vi "Construct Terminal Enabled State Binding.vi"(7 "Initial State (T)":bool=TRUE, 8 "FALSE State (Disabled and Grayed Out)":T1(ring)=enum."Disabled and Grayed Out", 9 "TRUE State (Enabled)":T1(ring), 10 "Control":refnum<vi>) -> (0 "error out":errorcluster, 3 "TerminalEnabledStateBinding":refnum<class "TerminalEnabledStateBinding.lvclass">)   [LabVIEW 2020, in "MVA Framework.lvlib" / "TerminalEnabledStateBinding.lvclass"]
doc: "构建终端启用状态绑定"
uses:
  TerminalEnabledStateBinding.lvclass
  TerminalPropertyBinding/TerminalPropertyBinding.lvclass/TerminalPropertyBinding.ctl
  TerminalEnabledStateBinding.lvclass/TerminalEnabledStateBinding.ctl
  TerminalPropertyBinding/TerminalPropertyBinding.lvclass
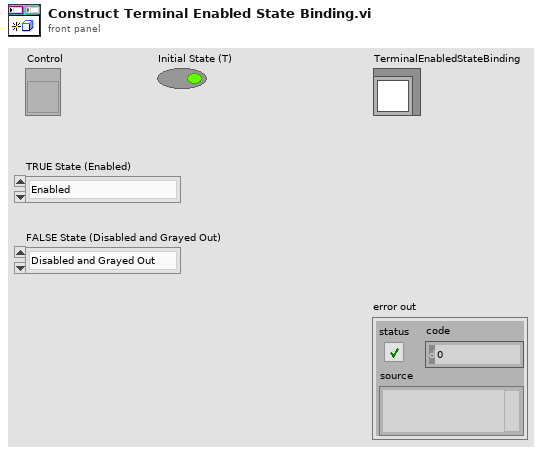
[diagram p1: front panel]
types:
  T1 = enum8{"Enabled", "Disabled", "Disabled and Grayed Out"}
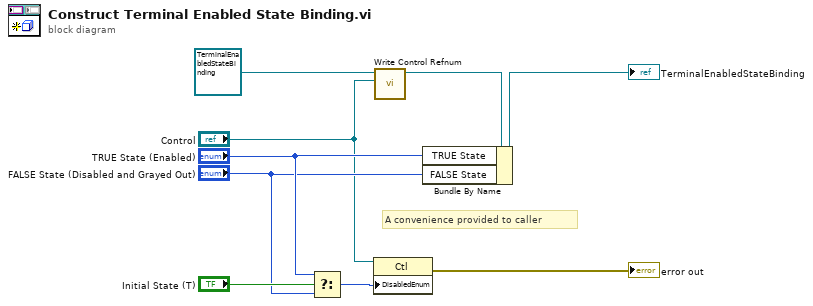
[diagram p0: block diagram]
diagram:
  # "A convenience provided to caller"
  n1 = Select(t="TRUE State (Enabled)", s="Initial State (T)", f="FALSE State (Disabled and Grayed Out)") -> (s? t:f=w4:T1)
  n2 = property class="Ctl"(reference="Control", "DisabledEnum"=w4) -> (error out=→"error out":errorcluster)  [unwired: 1 in, 1 out]
  n3 = call "Write Control Refnum.vi"("Ctl Refnum"="Control", "TerminalReference in"=refnum<class "TerminalEnabledStateBinding.lvclass"> refnum ("TerminalEnabledStateBinding.lvclass")) -> ("TerminalReferenceBinding Out"=w2:refnum<class "TerminalEnabledStateBinding.lvclass">)  [unwired: 9 in]
  n4 = Bundle By Name(cluster=w2, "TRUE State"="TRUE State (Enabled)", "FALSE State"="FALSE State (Disabled and Grayed Out)") -> (→"TerminalEnabledStateBinding":refnum<class "TerminalEnabledStateBinding.lvclass">)
